vi "check if start time tag is mapped.vi"(8 "error in":errorcluster, 10 "engine in":refnum<class "Engine Parent Editor Node.lvclass">, 11 "shared memory editor node in":refnum<class "module editor node.lvclass">) -> (0 "error out":errorcluster, 1 "start tag mapped?":bool, 2 "engine out":refnum<class "Engine Parent Editor Node.lvclass">, 3 "shared memory editor node out":refnum<class "module editor node.lvclass">)   [LabVIEW 2014, in "Shared Memory editor node.lvclass"]
uses:
  Shared Memory editor node.lvclass
  <vilib>/NI/DCAF/Tag Editor Core/Configuration Editor/Classes/Module editor node/module editor node.lvclass
  <vilib>/NI/DCAF/Tag Editor Core/Configuration Editor/Classes/Engine Parent/Engine Parent Editor Node.lvclass
  <vilib>/NI/Configuration Framework/serializable configuration/NISE_CEF_serializable configuration.lvclass/NISE_CEF_serializable configuration.ctl
  <vilib>/Utility/LVClass/Get LV Class Name.vi
  <vilib>/NI/Configuration Framework/error generator/NISE_error generator.vi
  <vilib>/NI/Module Execution Interface/Engine Configuration/engine configuration.lvclass
  <vilib>/NI/Configuration Framework/serializable configuration/NISE_CEF_serializable configuration.lvclass
  module/configuration/Shared Memory configuration.lvclass
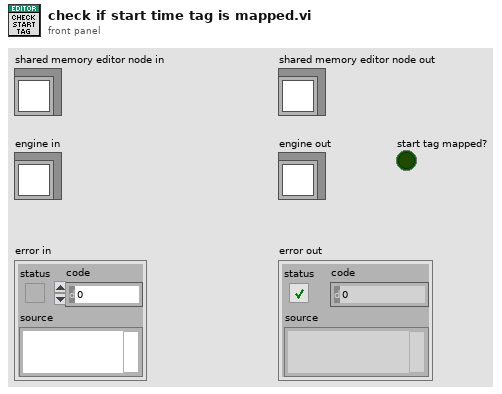
[diagram p1: front panel]
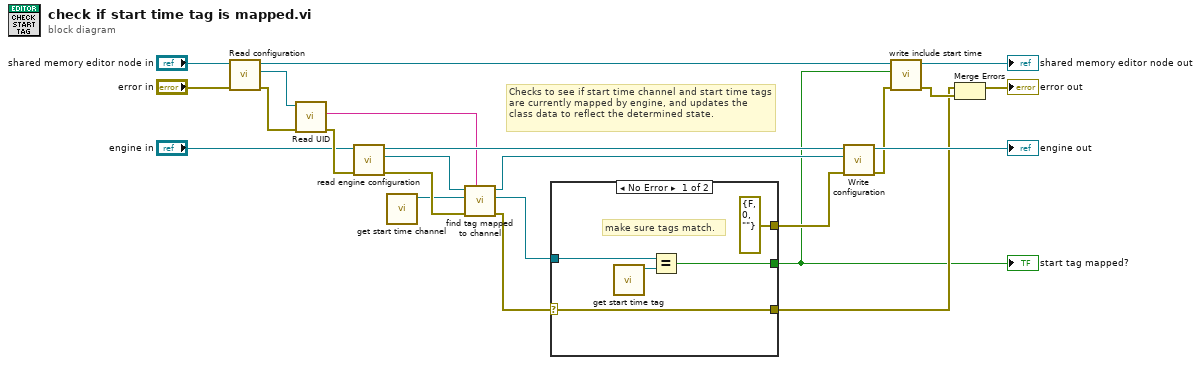
[diagram p0: block diagram]
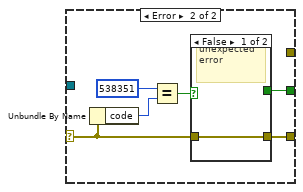
[diagram p2: hidden frame]
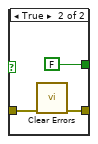
[diagram p3: hidden frame]
diagram:
  # "Checks to see if start time channel and start time tags are currently mapped by engine, and updates the class data to reflect the determined state."
  n1 = call-dynamic "Read configuration.vi"("error in"="error in", "NISE_CEF_serializable node in"="shared memory editor node in") -> ("error out"=w22:errorcluster, "configuration"=w23:refnum<class "NISE_CEF_serializable configuration.lvclass">, "NISE_CEF_serializable node out"=w14:refnum<class "module editor node.lvclass">)  [unwired: 7 in]
  n2 = call <vilib>:"Read UID.vi"("error in"=w22, "configuration in"=w23) -> ("error out"=w11:errorcluster, "instance id"=w4:string)  [unwired: 7 in, 1 out]
  n3 = call <vilib>:"read engine configuration.vi"("error in"=w11, "Engine Parent Editor Node in"="engine in") -> ("error out"=w9:errorcluster, "engine configuration"=w20:refnum<class "engine configuration.lvclass">, "Engine Parent Editor Node out"=w19:refnum<class "Engine Parent Editor Node.lvclass">)  [unwired: 7 in]
  n4 = call "get start time channel.vi"() -> ("channel"=w8:refnum<class "TBM channel.lvclass">)  [unwired: 11 in]
  n5 = call <vilib>:"find tag mapped to channel.vi"("owner"=w4, "error in"=w9, "channel"=w8, "engine configuration in"=w20) -> ("error out"=w16:errorcluster, "tag"=w15:refnum<class "tag descriptor.lvclass">, "engine configuration out"=w17:refnum<class "engine configuration.lvclass">)  [unwired: 5 in]
  n6 = case shown="No Error" w16 {
    selector: w16 -> [w25 w30]
    tunnel: [w28 w29] -> w1
    tunnel: [w25 w31] -> w3
    tunnel: w15 -> [w27 _]
    tunnel: [errorcluster {"status"=FALSE, "code"=0, "source"=""} ("error in") _] -> w2
    frame No Error {
      # "make sure tags match."
      n7 = call "get start time tag.vi"() -> ("tag"=w26:refnum<class "tag descriptor.lvclass">)  [unwired: 11 in]
      n8 = Equal?(x=w27, y=w26) -> (x = y?=w28:bool)
    }
    frame Error {
      n9 = Unbundle By Name(w30) -> ("code"=w32:i32)
      n10 = Equal?(x=538351, y=w32) -> (x = y?=w33:bool)
      n11 = case shown="False" w33 {
        tunnel: w30 -> [w35 w38]
        tunnel: [w35 w37] -> w31
        tunnel: [_ FALSE] -> w29
        frame False {
          # "unexpected\nerror"
        }
        frame True {
          n12 = call <vilib>:"Clear Errors.vi"("error in (no error)"=w38) -> ("error out"=w37:errorcluster)  [unwired: 5 in, 1 out]
        }
      }
    }
  }
  "start tag mapped?" <- w1
  n13 = call-dynamic "Write configuration.vi"("error in"=w2, "configuration"=w17, "NISE_CEF_serializable node in"=w19) -> ("error out"=w5:errorcluster, "NISE_CEF_serializable node out"=→"engine out":refnum<class "Engine Parent Editor Node.lvclass">)  [unwired: 7 in]
  n14 = call "write include start time.vi"("error in"=w5, "include start time"=w1, "shared memory editor node"=w14) -> ("error out"=w6:errorcluster, "shared memory editor node out"=→"shared memory editor node out":refnum<class "module editor node.lvclass">)  [unwired: 7 in]
  n15 = Merge Errors(w3, w6) -> (→"error out":errorcluster)
